vi "TCP multiple open.vi"(2 "timeout ms (60000)":i32=300, 3 "Ports":string[](array[string]), 4 "error in 1 (no error)":errorcluster, 5 "IP Addresses":string[](array[string])) -> (0 "error out":errorcluster, 1 "Array":refnum<k5>[](array[refnum]))   [LabVIEW 2013]
panel:
  out "Open Errors":errorcluster[](array[cluster])
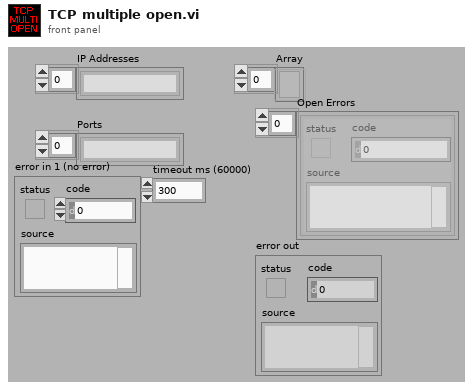
[diagram p1: front panel]
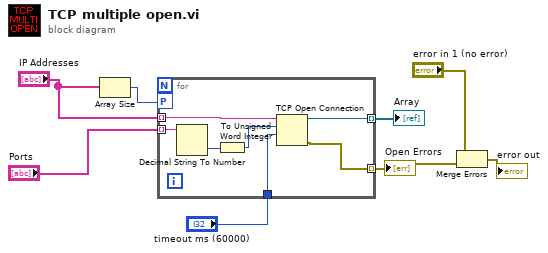
[diagram p0: block diagram]
diagram:
  n1 = Array Size(array="IP Addresses") -> (size(s)=w5:i32)
  n2 = for {
    workers-P: w5 -> [_]
    tunnel: "IP Addresses" -> [w15] mode=indexing
    tunnel: "Ports" -> [w14] mode=indexing
    tunnel: [w13] -> w8 mode=indexing
    tunnel: [w11] -> w3 mode=indexing
    tunnel: "timeout ms (60000)" -> [w9]
    n3 = Decimal String To Number(string=w14) -> (number=w12:i32)  [unwired: 2 in, 1 out]
    n4 = To Unsigned Word Integer(number=w12) -> (unsigned 16bit integer=w10:u16)
    n5 = TCP Open Connection(address=w15, remote port or service name=w10, timeout ms (60000)=w9) -> (connection ID=w13:refnum<k5>, error out=w11:errorcluster)  [unwired: 2 in]
  }
  "Array" <- w8
  "Open Errors" <- w3
  n6 = Merge Errors("error in 1 (no error)", w3) -> (→"error out":errorcluster)
